vi "Post Status.vi"(8 "error in (no error)":errorcluster, 10 "Status Message":string) -> (0 "error out":errorcluster)   [LabVIEW 2016, in "Hall Effect Library.lvlib"]
uses:
  Hall Effect Library.lvlib
  Public/Controls/Message Types.ctl
  Global Variables/Communication.vi
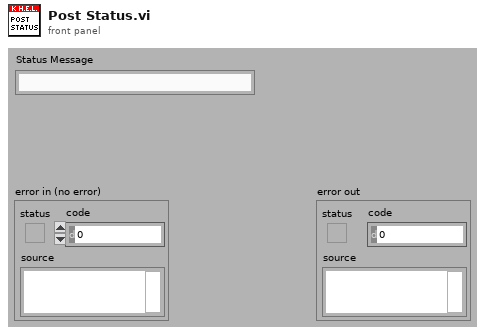
[diagram p1: front panel]
types:
  T1 = typedef "Hall Effect Library.lvlib/Message Types.ctl" = enum16{"Status", "New Data", "Test End Normal", "Test End User Abort", "Test End Error"}
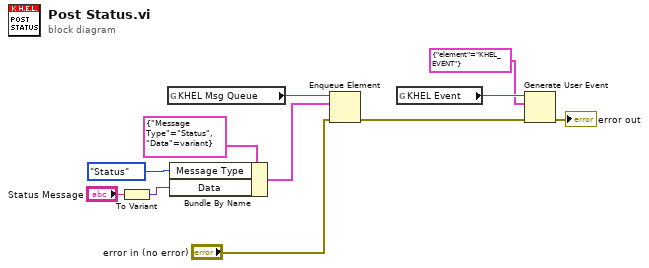
[diagram p0: block diagram]
diagram:
  n1 = To Variant(anything="Status Message") -> (Variant=w7:variant)
  n2 = global read "Communication.vi" "KHEL Msg Queue"() -> (w11:refnum<queue>)
  n3 = Bundle By Name(cluster=cluster{"Message Type":T1, "Data":variant} {"Message Type"=enum."Status", "Data"=variant} ("element"), "Message Type"=Message_Types."Status", "Data"=w7) -> (w6:cluster{"Message Type":T1, "Data":variant})
  n4 = Enqueue Element(queue=w11, element=w6, error in (no error)="error in (no error)") -> (error out=w4:errorcluster)  [unwired: 3 out]
  n5 = global read "Communication.vi" "KHEL Event"() -> (w2:refnum<user-event>)
  n6 = Generate User Event(user event=w2, event data cluster=cluster{"element":string} {"element"="KHEL_EVENT"}, error in=w4) -> (error out=→"error out":errorcluster)  [unwired: 1 in, 1 out]
